vi "Cypher Lithography 2.0_Feng_MFP3D_Lucy.vi"(0 "Nodes on the line\n(  x      ,       y   )":dbl[][](array[numeric])=[[-5e-06, -5e-06], [5e-06, 5e-06]] min=-4.5e-05 max=4.5e-05 step=1e-09 format="%#_6pm", 1 "V":dbl[](array[numeric]), 2 "Litho Speed":dbl=5e-07 format="%#_6pm/s", 3 "Z SetPoint":dbl format="%#_6p", 4 "New nodes spacing":dbl=1e-06 format="%#_6pm", 5 "display wave":bool, 6 "Need interpolate new nodes?":bool, 7 "PID close":bool) -> ()   [LabVIEW 2016]
uses:
  Cypher XY LVDT Parameters_MFP3D_Lucy.vi
  <vilib>/Utility/file.llb/Write To Spreadsheet File (DBL).vi
panel:
  out "error out":errorcluster
  out "XY Graph":T1(graph)
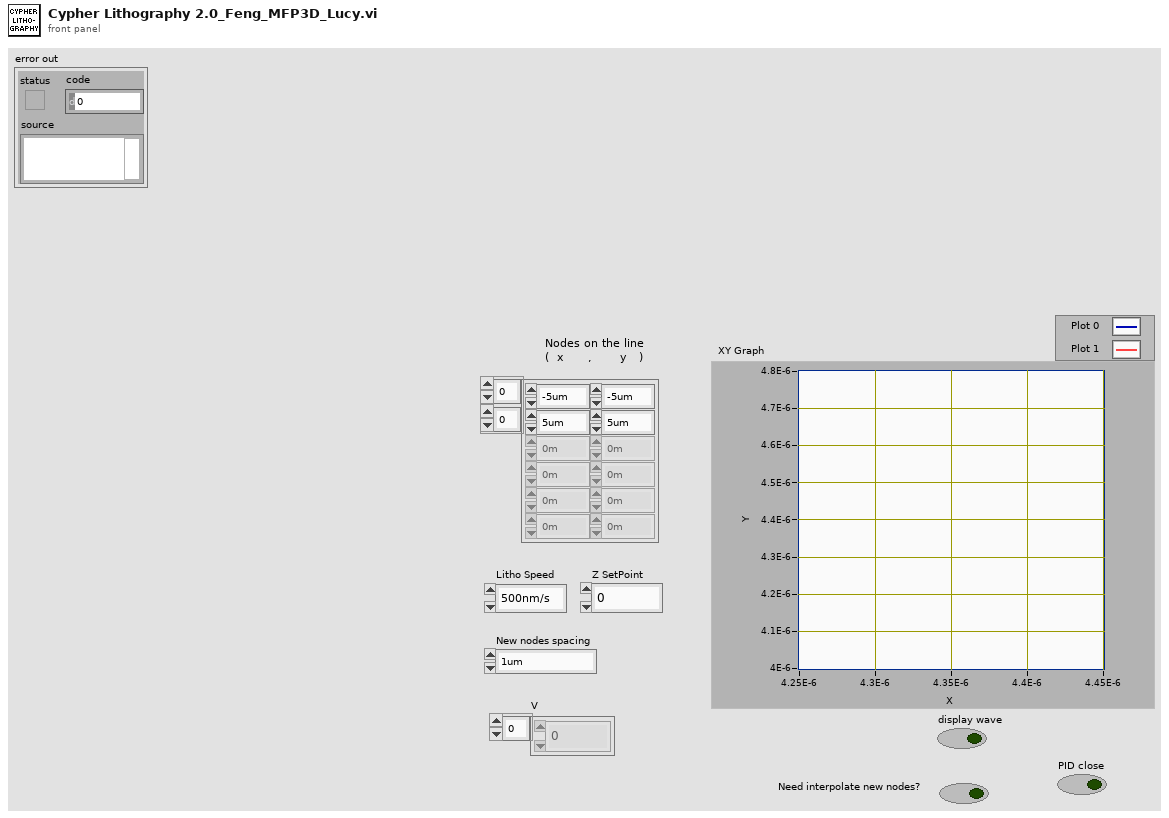
[diagram p1: front panel]
types:
  T1 = cluster{"Nodes on the line\n(  x      ,       y   )":dbl[], "Nodes on the line\n(  x      ,       y   )":dbl[]}[]
  T2 = cluster{"Interpolate result":dbl[], "Interpolate result":dbl[]}
  T3 = enum16{"open", "replace", "create", "open or create", "replace or create", "replace or create with confirmation"}
  T4 = cluster{"Nodes on the line\n(  x      ,       y   )":dbl[], "Nodes on the line\n(  x      ,       y   )":dbl[]}
  T5 = cluster{"Interpolate result":dbl[], "Interpolate result":dbl[]}[]
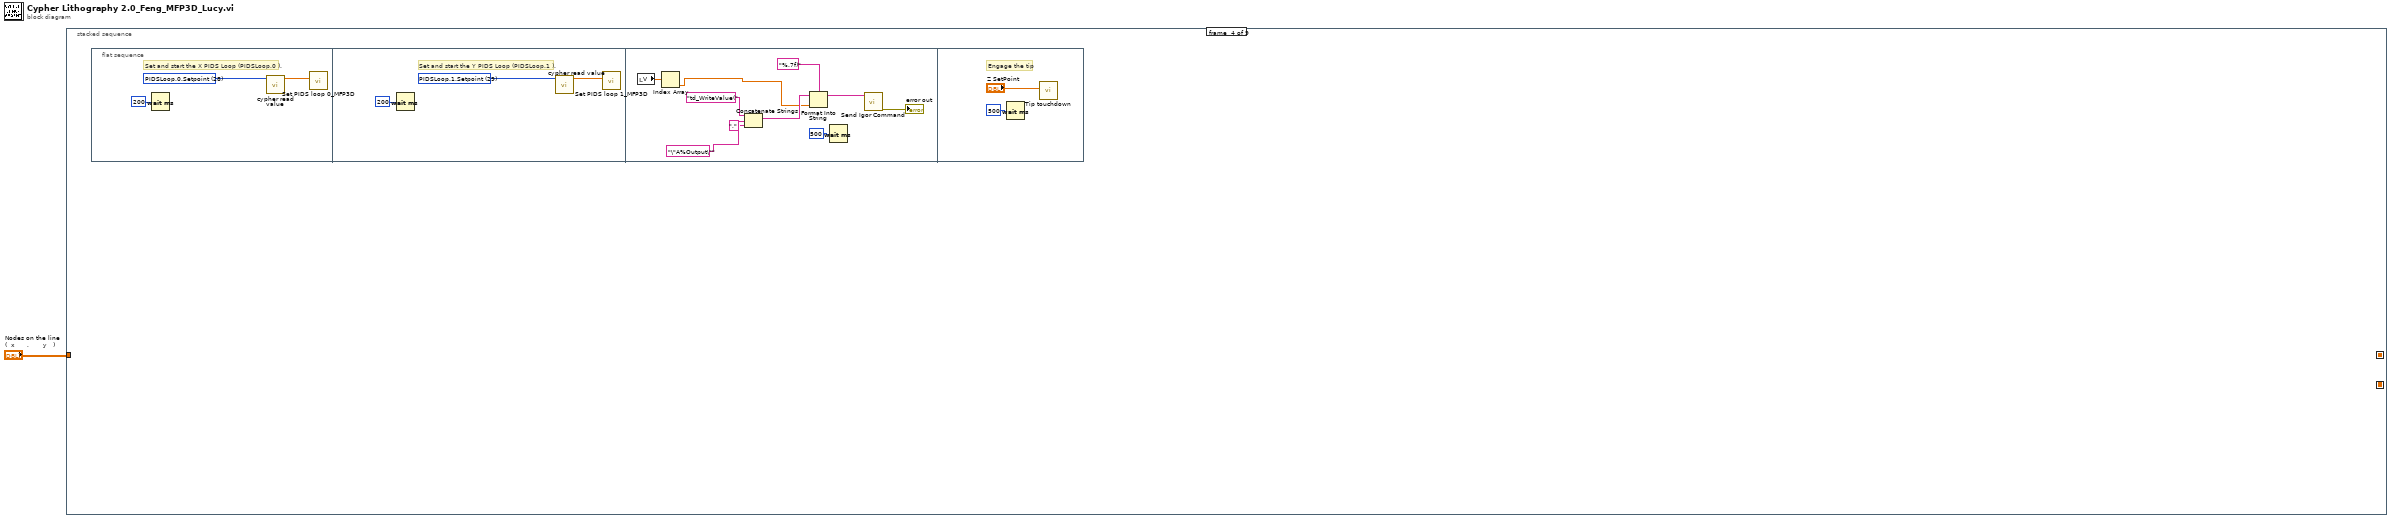
[diagram p0: block diagram]
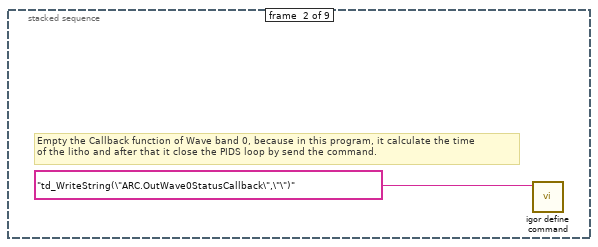
[diagram p3: hidden frame]
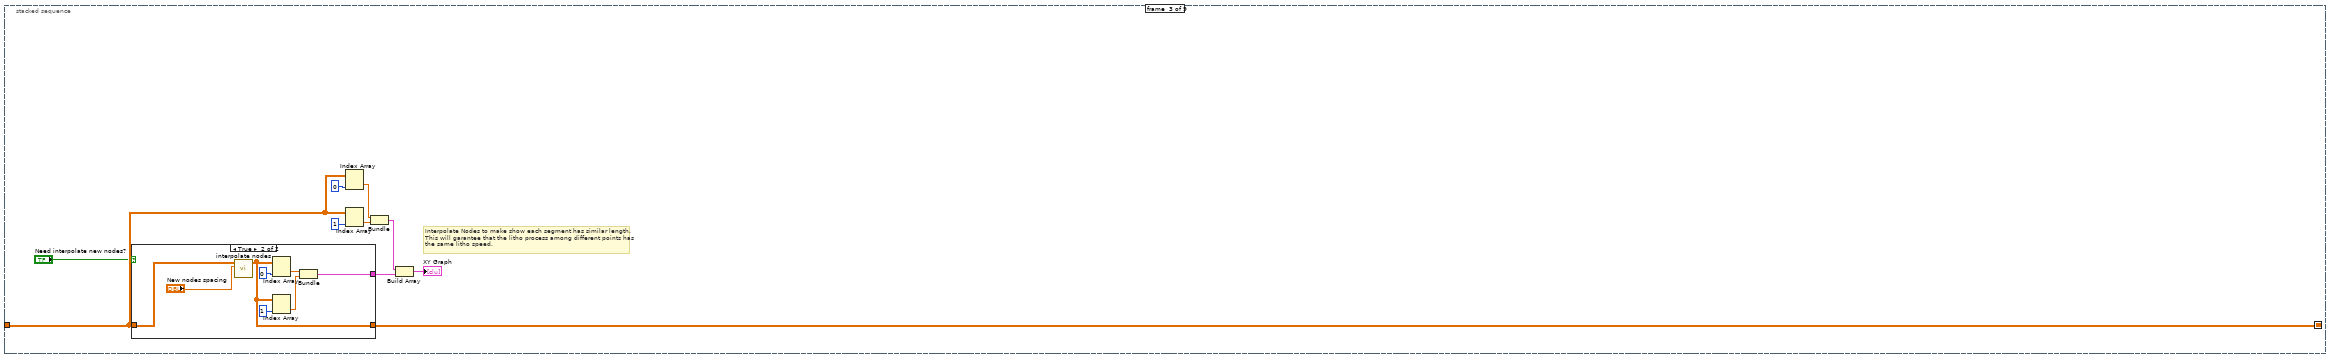
[diagram p4: hidden frame]
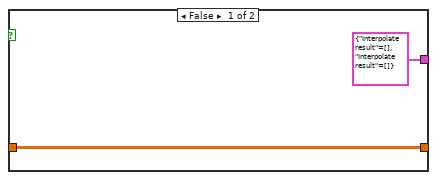
[diagram p5: hidden frame]
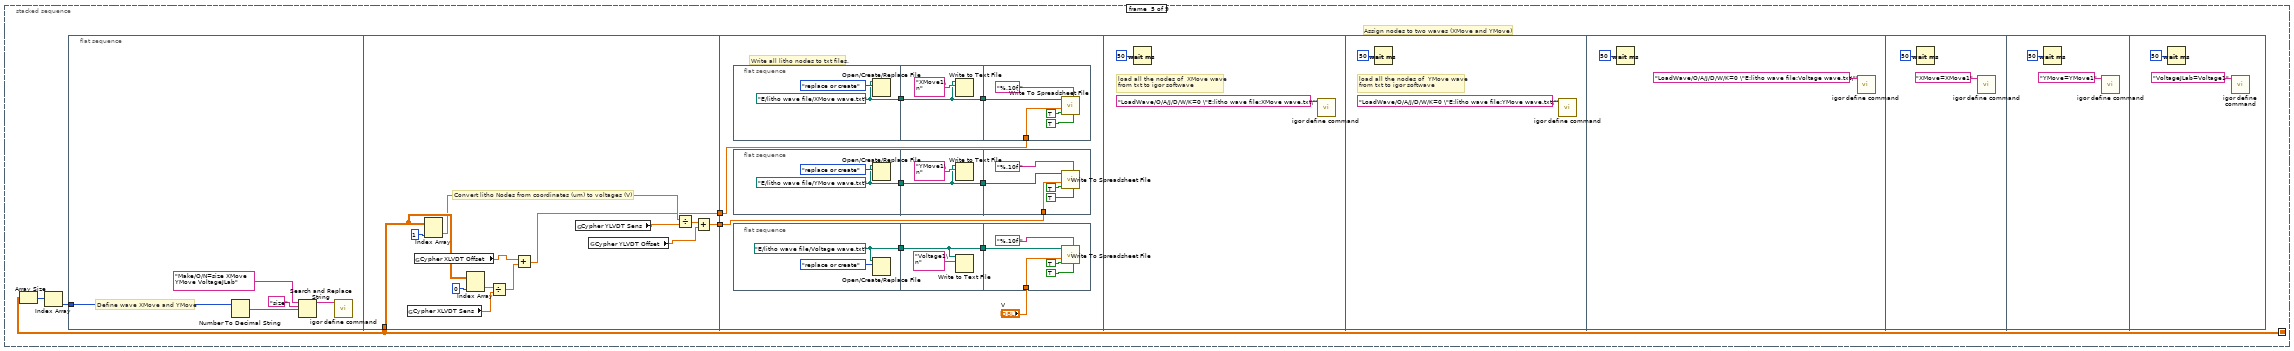
[diagram p6: hidden frame]
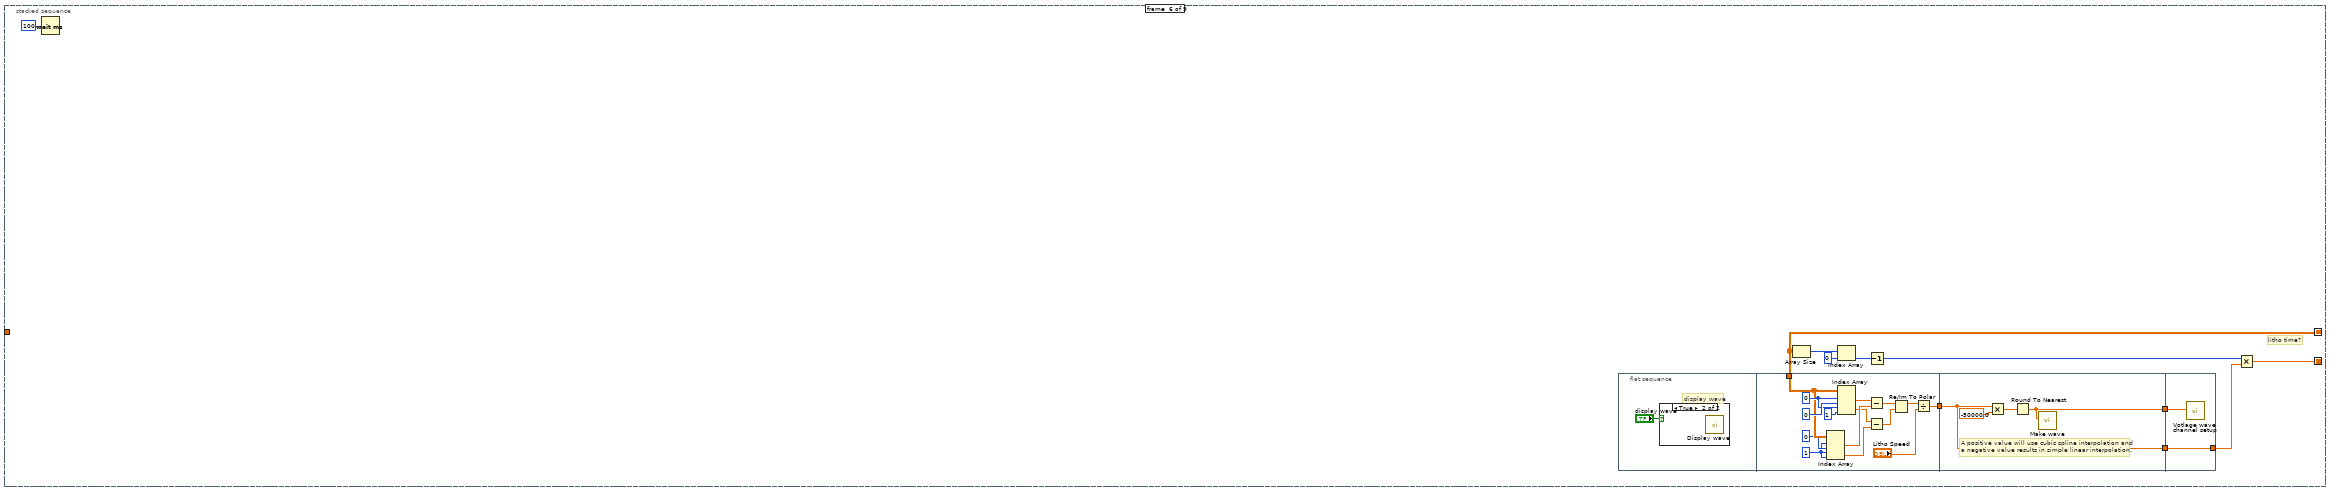
[diagram p7: hidden frame]
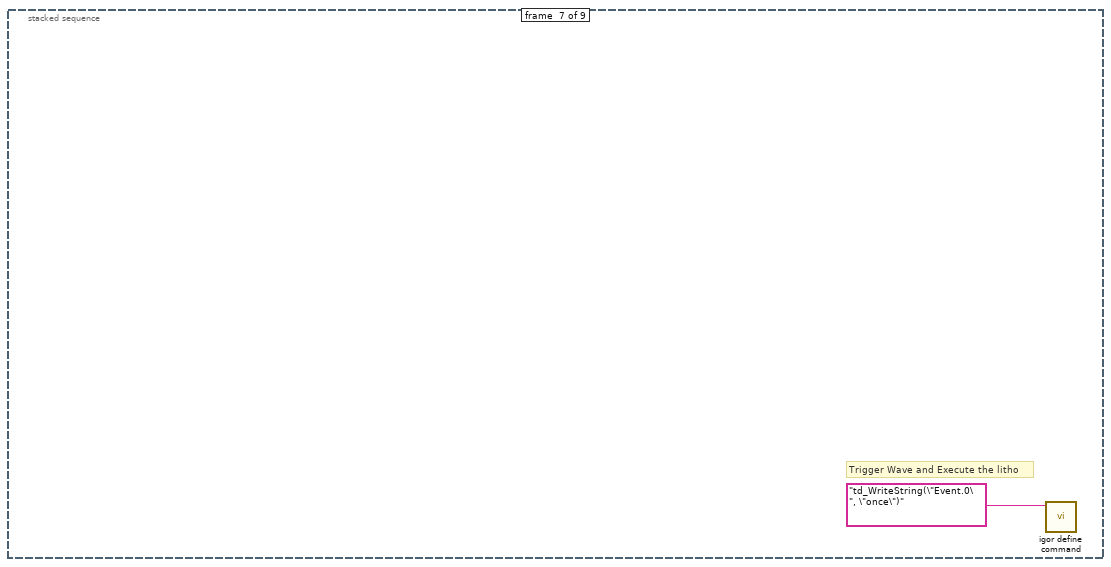
[diagram p9: hidden frame]
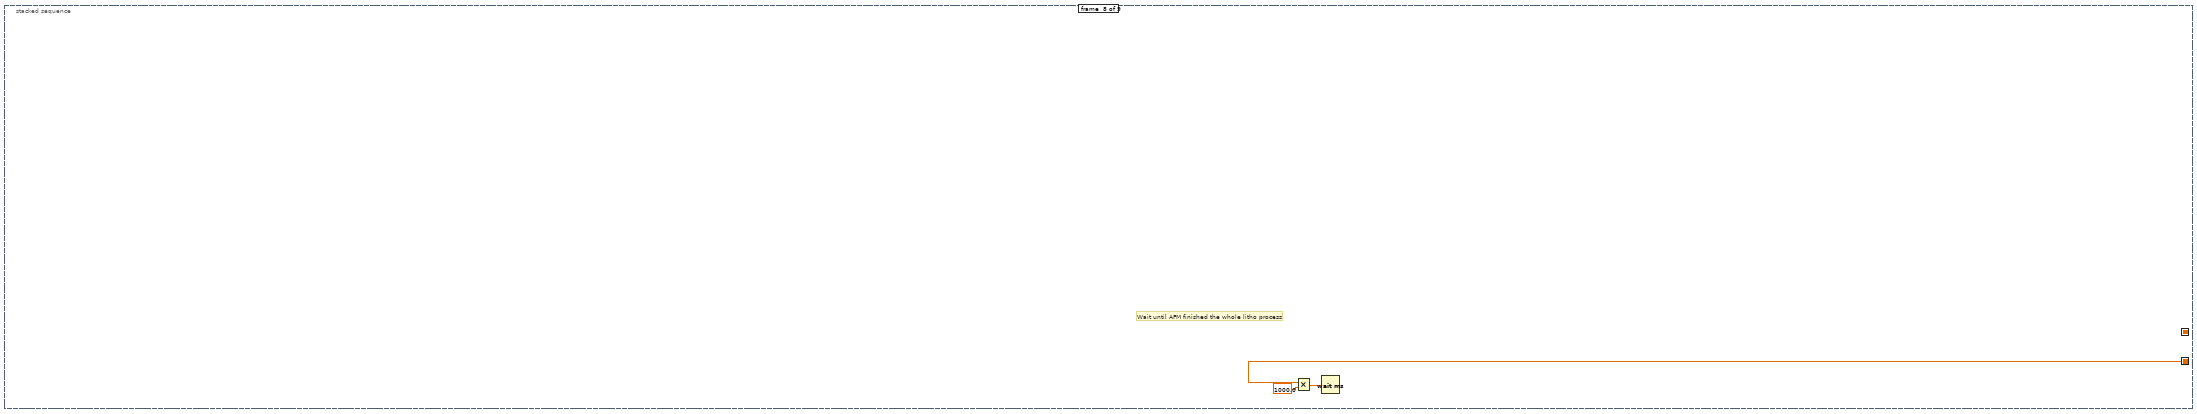
[diagram p10: hidden frame]
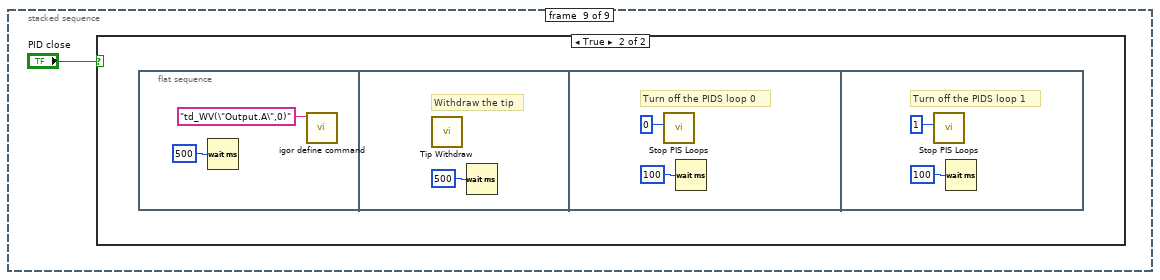
[diagram p11: hidden frame]
diagram:
  n1 = stacked-sequence {
    seq-local: [_ _ w4 _ _ _ _ _ _] -> [_ _ _ _ w42 w121 _ _ _]
    seq-local: [_ _ _ _ _ w117 _ _ _] -> [_ _ _ _ _ _ _ w148 _]
    tunnel: "Nodes on the line\n(  x      ,       y   )" -> [_ _ w6 _ _ _ _ _ _]
    frame #0 {
    }
    frame #1 {
      # "Empty the Callback function of Wave band 0, because in this program, it calculate the time \nof the litho and after that it close the PIDS loop by send the command."
      n2 = call "igor define command.vi"("Command"="td_WriteString(\"ARC.OutWave0StatusCallback\",\"\")") -> ()  [unwired: 11 out]
    }
    frame #2 {
      # "Interpolate Nodes to make show each segment has similar length.\nThis will garantee that the litho process among different points has\nthe same litho speed."
      n3 = case shown="True" "Need interpolate new nodes?" {
        tunnel: w6 -> [w14 w22]
        tunnel: [T2 {"Interpolate result"=[], "Interpolate result"=[]} w17] -> w5
        tunnel: [w14 w16] -> w4
        frame False {
        }
        frame True {
          n4 = call "interpolate nodes.vi"("Interpolate spacing"="New nodes spacing", "Nodes on the line\n(  x      ,       y   )"=w22) -> ("Interpolate result"=w16:dbl[][])  [unwired: 9 in]
          n5 = Index Array(array=w16, index (col)=0 ("disabled index (col)")) -> (element=w19:dbl[])  [unwired: 1 in]
          n6 = Index Array(array=w16, index (col)=1 ("disabled index (col)")) -> (element=w18:dbl[])  [unwired: 1 in]
          n7 = Bundle("Interpolate result"=w19, "Interpolate result"=w18) -> (w17:T2)  [unwired: 1 in]
        }
      }
      n8 = Index Array(array=w6, index (col)=0 ("disabled index (col)")) -> (element=w11:dbl[])  [unwired: 1 in]
      n9 = Index Array(array=w6, index (col)=1 ("disabled index (col)")) -> (element=w9:dbl[])  [unwired: 1 in]
      n10 = Bundle("Nodes on the line\n(  x      ,       y   )"=w11, "Nodes on the line\n(  x      ,       y   )"=w9) -> (w8:T4)  [unwired: 1 in]
      n11 = Build Array(w8, w5) -> (→"XY Graph":T5)
    }
    frame #3 {
      n12 = flat-sequence {
        frame #0 {
          w24 = u16 28 items=["XSensor", "YSensor", "ZSensor", "InA", "InB", "InFast", "In_Amplitude1", "In_Amplitude2", "In_Phase1", "In_Phase2", "PiezoX", "PiezoY", "PiezoZ", "OutA", "OutB", "OutC", "DDS_Frequency1", "DDS_Frequency2", "DDS_Amplitude1", "DDS_Amplitude2", "DDS_DCOffset", "Laser_Sum", "Laser_Difference", "Laser_Lateral", "XLVDT Sensitivity", "YLVDT Sensitivity", "XLVDT Offset", "YLVDT Offset", "PIDSLoop.0.Setpoint", "PIDSLoop.1.Setpoint"] ("Input")
          # "Set and start the X PIDS Loop (PIDSLoop.0 )."
          n13 = Wait (ms)(milliseconds to wait=u32 200) -> ()  [unwired: 1 out]
          n14 = call "cypher read value.vi"("Input"=w24) -> ("Result"=w25:dbl)  [unwired: 10 in]
          n15 = call "Set PIDS loop 0_MFP3D.vi"("X  Setpoint"=w25) -> ()  [unwired: 11 in]
        }
        frame #1 {
          w27 = u16 29 items=["XSensor", "YSensor", "ZSensor", "InA", "InB", "InFast", "In_Amplitude1", "In_Amplitude2", "In_Phase1", "In_Phase2", "PiezoX", "PiezoY", "PiezoZ", "OutA", "OutB", "OutC", "DDS_Frequency1", "DDS_Frequency2", "DDS_Amplitude1", "DDS_Amplitude2", "DDS_DCOffset", "Laser_Sum", "Laser_Difference", "Laser_Lateral", "XLVDT Sensitivity", "YLVDT Sensitivity", "XLVDT Offset", "YLVDT Offset", "PIDSLoop.0.Setpoint", "PIDSLoop.1.Setpoint"] ("Input")
          # "Set and start the Y PIDS Loop (PIDSLoop.1 )."
          n16 = Wait (ms)(milliseconds to wait=u32 200) -> ()  [unwired: 1 out]
          n17 = call "cypher read value.vi"("Input"=w27) -> ("Result"=w28:dbl)  [unwired: 10 in]
          n18 = call "Set PIDS loop 1_MFP3D.vi"("Y Setpoint"=w28) -> ()  [unwired: 11 in]
        }
        frame #2 {
          n19 = local read "V"() -> (w38:dbl[])
          n20 = Index Array(array=w38) -> (element=w30:dbl)  [unwired: 1 in]
          n21 = Concatenate Strings("td_WriteValue(", "\"A%Output\"", "," ("string")) -> (w33:string)
          n22 = Format Into String "Format Into String"(format string="%.7f)" ("Number resolutio"), initial string=w33, w30) -> (resulting string=w35:string)  [unwired: 1 in, 1 out]
          n23 = Wait (ms)(milliseconds to wait=u32 500) -> ()  [unwired: 1 out]
          n24 = call <vilib>:"Send Igor Command.vi"("Command"=w35) -> ("error out"=→"error out":errorcluster)  [unwired: 7 in, 2 out]
        }
        frame #3 {
          # "Engage the tip"
          n25 = Wait (ms)(milliseconds to wait=u32 500) -> ()  [unwired: 1 out]
          n26 = call "Tip touchdown.vi"("Z SetPoint"="Z SetPoint") -> ()  [unwired: 11 out]
        }
      }
    }
    frame #4 {
      # "Assign nodes to two waves (XMove and YMove)"
      n27 = Array Size(array=w42) -> (size(s)=w43:i32[])
      n28 = Index Array(array=w43) -> (element=w41:i32)  [unwired: 1 in]
      n29 = flat-sequence {
        tunnel: w41 -> [w46]
        tunnel: w42 -> [w60]
        tunnel: [w56] -> w45
        tunnel: [w55] -> w44
        tunnel: w45 -> [w68]
        tunnel: w44 -> [w67]
        frame #0 {
          # "Define wave XMove and YMove"
          n30 = Number To Decimal String(number=w46) -> (decimal integer string=w48:string)  [unwired: 1 in]
          n31 = Search and Replace String(input string="Make/O/N=size XMove YMove VoltageJLab", search string="size", replace string=w48) -> (result string=w47:string)  [unwired: 1 in, 7 out]
          n32 = call "igor define command.vi"("Command"=w47) -> ()  [unwired: 11 out]
        }
        frame #1 {
          # "Convert litho Nodes from coordinates (um) to voltages (V)"
          n33 = global read "Cypher XY LVDT Parameters_MFP3D_Lucy.vi" "Cypher XLVDT Sens"() -> (w53:dbl)
          n34 = global read "Cypher XY LVDT Parameters_MFP3D_Lucy.vi" "Cypher XLVDT Offset"() -> (w54:dbl)
          n35 = Index Array(array=w60, index (col)=1 ("disabled index (col)")) -> (element=w57:dbl[])  [unwired: 1 in]
          n36 = Index Array(array=w60, index (col)=0 ("disabled index (col)")) -> (element=w58:dbl[])  [unwired: 1 in]
          n37 = Divide(x=w58, y=w53) -> (x/y=w62:dbl[])
          n38 = Add(x=w54, y=w62) -> (x+y=w55:dbl[])
          n39 = global read "Cypher XY LVDT Parameters_MFP3D_Lucy.vi" "Cypher YLVDT Sens"() -> (w52:dbl)
          n40 = global read "Cypher XY LVDT Parameters_MFP3D_Lucy.vi" "Cypher YLVDT Offset"() -> (w51:dbl)
          n41 = Divide(x=w57, y=w52) -> (x/y=w61:dbl[])
          n42 = Add(x=w61, y=w51) -> (x+y=w56:dbl[])
        }
        frame #2 {
          # "Write all litho nodes to txt files."
          n43 = flat-sequence {
            tunnel: [w91] -> w72
            tunnel: w72 -> [w93]
            tunnel: [w93] -> w71
            tunnel: w71 -> [w97]
            tunnel: w67 -> [w96]
            frame #0 {
              w91 = path "E:/litho wave file/XMove wave.txt" ("\"XMove wave\" file path")
              n44 = Open/Create/Replace File(file path (use dialog)=w91, operation (0:open)=T3."replace or create") -> ()  [unwired: 4 in, 3 out]
            }
            frame #1 {
              n45 = Write to Text File(file (use dialog)=w93, text="XMove1\n") -> ()  [unwired: 2 in, 3 out]
            }
            frame #2 {
              n46 = call-poly <vilib>:"Write To Spreadsheet File.vi"("transpose? (no:F)"=TRUE, "format (%.3f)"="%.10f ", "append to file? (new file:F)"=TRUE, "1D data"=w96, "file path (dialog if empty)"=w97) -> ()  [unwired: 3 in, 1 out]
            }
          }
          n47 = flat-sequence {
            tunnel: [w82] -> w70
            tunnel: w70 -> [w84]
            tunnel: [w84] -> w69
            tunnel: w69 -> [w88]
            tunnel: w68 -> [w87]
            frame #0 {
              w82 = path "E:/litho wave file/YMove wave.txt" ("\"YMove wave\" file path")
              n48 = Open/Create/Replace File(file path (use dialog)=w82, operation (0:open)=T3."replace or create") -> ()  [unwired: 4 in, 3 out]
            }
            frame #1 {
              n49 = Write to Text File(file (use dialog)=w84, text="YMove1\n") -> ()  [unwired: 2 in, 3 out]
            }
            frame #2 {
              n50 = call-poly <vilib>:"Write To Spreadsheet File.vi"("transpose? (no:F)"=TRUE, "format (%.3f)"="%.10f ", "append to file? (new file:F)"=TRUE, "1D data"=w87, "file path (dialog if empty)"=w88) -> ()  [unwired: 3 in, 1 out]
            }
          }
          n51 = flat-sequence {
            tunnel: [w73] -> w66
            tunnel: w66 -> [w75]
            tunnel: [w75] -> w65
            tunnel: w65 -> [w79]
            tunnel: "V" -> [w77]
            frame #0 {
              w73 = path "E:/litho wave file/Voltage wave.txt" ("file path (use dialog)")
              n52 = Open/Create/Replace File(file path (use dialog)=w73, operation (0:open)=T3."replace or create") -> ()  [unwired: 4 in, 3 out]
            }
            frame #1 {
              n53 = Write to Text File(file (use dialog)=w75, text="Voltage1\n") -> ()  [unwired: 2 in, 3 out]
            }
            frame #2 {
              n54 = call-poly <vilib>:"Write To Spreadsheet File.vi"("transpose? (no:F)"=TRUE, "format (%.3f)"="%.10f ", "append to file? (new file:F)"=TRUE, "1D data"=w77, "file path (dialog if empty)"=w79) -> ()  [unwired: 3 in, 1 out]
            }
          }
        }
        frame #3 {
          # "load all the nodes of  XMove wave\nfrom txt to igor softwave"
          n55 = Wait (ms)(milliseconds to wait=u32 50) -> ()  [unwired: 1 out]
          n56 = call "igor define command.vi"("Command"="LoadWave/O/A/J/D/W/K=0 \"E:litho wave file:XMove wave.txt\"") -> ()  [unwired: 11 out]
        }
        frame #4 {
          # "load all the nodes of  YMove wave\nfrom txt to igor softwave"
          n57 = Wait (ms)(milliseconds to wait=u32 50) -> ()  [unwired: 1 out]
          n58 = call "igor define command.vi"("Command"="LoadWave/O/A/J/D/W/K=0 \"E:litho wave file:YMove wave.txt\"") -> ()  [unwired: 11 out]
        }
        frame #5 {
          n59 = Wait (ms)(milliseconds to wait=u32 50) -> ()  [unwired: 1 out]
          n60 = call "igor define command.vi"("Command"="LoadWave/O/A/J/D/W/K=0 \"E:litho wave file:Voltage wave.txt\"") -> ()  [unwired: 11 out]
        }
        frame #6 {
          n61 = Wait (ms)(milliseconds to wait=u32 50) -> ()  [unwired: 1 out]
          n62 = call "igor define command.vi"("Command"="XMove=XMove1") -> ()  [unwired: 11 out]
        }
        frame #7 {
          n63 = Wait (ms)(milliseconds to wait=u32 50) -> ()  [unwired: 1 out]
          n64 = call "igor define command.vi"("Command"="YMove=YMove1") -> ()  [unwired: 11 out]
        }
        frame #8 {
          n65 = Wait (ms)(milliseconds to wait=u32 50) -> ()  [unwired: 1 out]
          n66 = call "igor define command.vi"("Command"="VoltageJLab=Voltage1") -> ()  [unwired: 11 out]
        }
      }
    }
    frame #5 {
      # "litho time?"
      n67 = Wait (ms)(milliseconds to wait=u32 100) -> ()  [unwired: 1 out]
      n68 = flat-sequence {
        tunnel: w121 -> [w135]
        tunnel: [w124] -> w122
        tunnel: w122 -> [w140]
        tunnel: [w140] -> w113
        tunnel: [w139] -> w112
        tunnel: [w144] -> w118
        tunnel: w113 -> [w144]
        tunnel: w112 -> [w143]
        frame #0 {
          # "display wave"
          n69 = case shown="True" "display wave" {
            frame False {
            }
            frame True {
              n70 = call "Display wave.vi"() -> ()  [unwired: 1 out]
            }
          }
        }
        frame #1 {
          w133 = 1 ("index (row)")
          w137 = 0 ("index (row)")
          n71 = Index Array(array=w135, index (row) #1=w133, index (col) #1=0 ("disabled index (col)"), index (row) #2=w133, index (col) #2=w133) -> (element #1=w131:dbl, element #2=w130:dbl)
          n72 = Index Array(array=w135, index (row) #1=w137, index (col) #1=0 ("disabled index (col)"), index (row) #2=w137, index (col) #2=1 ("disabled index (col)")) -> (element #1=w132:dbl, element #2=w129:dbl)
          n73 = Subtract(x=w132, y=w131) -> (x-y=w128:dbl)
          n74 = Subtract(x=w129, y=w130) -> (x-y=w127:dbl)
          n75 = Re/Im To Polar(2:w127, 3:w128) -> (1:w126:dbl)  [unwired: 1 out]
          n76 = Divide(x=w126, y="Litho Speed") -> (x/y=w124:dbl)
        }
        frame #2 {
          # "A positive value will use cubic spline interpolation and \na negative value results in simple linear interpolation."
          n77 = Multiply(x=w140, y=-50000.0) -> (x*y=w141:dbl)
          n78 = Round To Nearest(number=w141) -> (nearest integer value=w139:dbl)
          n79 = call "Make wave.vi"("Totalpoints"=w139) -> ()  [unwired: 11 out]
        }
        frame #3 {
          n80 = call "Votlage wave channel setup.vi"("Totalpoints"=w143) -> ()  [unwired: 11 in]
        }
      }
      n81 = Array Size(array=w121) -> (size(s)=w120:i32[])
      n82 = Index Array(array=w120, index=0) -> (element=w116:i32)
      n83 = Decrement(x=w116) -> (x-1=w115:i32)
      n84 = Multiply(x=w115, y=w118) -> (x*y=w117:dbl)
    }
    frame #6 {
      # "Trigger Wave and Execute the litho"
      n85 = call "igor define command.vi"("Command"="td_WriteString(\"Event.0\", \"once\")") -> ()  [unwired: 11 out]
    }
    frame #7 {
      # "Wait until AFM finished the whole litho process"
      n86 = Multiply(x=w148, y=1000.0) -> (x*y=w146:dbl)
      n87 = Wait (ms)(milliseconds to wait=w146) -> ()  [unwired: 1 out]
    }
    frame #8 {
      n88 = case shown="True" "PID close" {
        frame False {
        }
        frame True {
          n89 = flat-sequence {
            frame #0 {
              n90 = Wait (ms)(milliseconds to wait=u32 500) -> ()  [unwired: 1 out]
              n91 = call "igor define command.vi"("Command"="td_WV(\"Output.A\",0)") -> ()  [unwired: 11 out]
            }
            frame #1 {
              # "Withdraw the tip"
              n92 = call "Tip Withdraw.vi"() -> ()  [unwired: 1 in]
              n93 = Wait (ms)(milliseconds to wait=u32 500) -> ()  [unwired: 1 out]
            }
            frame #2 {
              # "Turn off the PIDS loop 0"
              n94 = call "Stop PIS Loops.vi"("PIS Loop Number (0-5)"=u32 0) -> ()  [unwired: 11 out]
              n95 = Wait (ms)(milliseconds to wait=u32 100) -> ()  [unwired: 1 out]
            }
            frame #3 {
              # "Turn off the PIDS loop 1"
              n96 = call "Stop PIS Loops.vi"("PIS Loop Number (0-5)"=u32 1) -> ()  [unwired: 11 out]
              n97 = Wait (ms)(milliseconds to wait=u32 100) -> ()  [unwired: 1 out]
            }
          }
        }
      }
    }
  }
